vi "LogScales.vi"() -> ()   [LabVIEW 2013]
uses:
  <vilib>/Heliosphere Research LLC/Advanced Plotting Toolkit/api_core/NewPlotScales.ctl
  <vilib>/Heliosphere Research LLC/Advanced Plotting Toolkit/api_plotting/LineProperties.ctl
  <vilib>/Heliosphere Research LLC/Advanced Plotting Toolkit/properties/Line.ctl
  <vilib>/Heliosphere Research LLC/Advanced Plotting Toolkit/properties/Line_Style.ctl
  <vilib>/Heliosphere Research LLC/Advanced Plotting Toolkit/typedefs/PlotColor.ctl
  <vilib>/Heliosphere Research LLC/Advanced Plotting Toolkit/properties/Marker.ctl
  <vilib>/Heliosphere Research LLC/Advanced Plotting Toolkit/properties/Marker_Style.ctl
  <vilib>/Heliosphere Research LLC/Advanced Plotting Toolkit/properties/Display.ctl
  <vilib>/Heliosphere Research LLC/Advanced Plotting Toolkit/Advanced Plotting Toolkit.lvlib
panel:
  in  "Y Axis Scale":T1
  in  "X Axis Scale":T1
  in  "Show Grid Lines":bool=TRUE
  out "Log Plot":picture
  # "Log Scales"
  # "When plotting data that spans several orders of magnitude, it's\noften useful to display the X or Y axes using a log scale.\n\nThe Toolkit provides two mechanisms for this.  Scales of type\n\"Log\" are displayed in the traditional fashion, using base 10.\nTry changing the Y scale, below.\n\nThe second mechanism is \"Symlog\" or symmetric log.  This\nscale type displays both positive and negative values; since\nzero cannot be displayed on a log scale, a small region around\nthe origin will use a linear scale.\n\nTry changing the X scale, below.  In Log mode, only positive\nvalues are displayed.  In Symlog mode, both positive and\nnegative values are displayed."
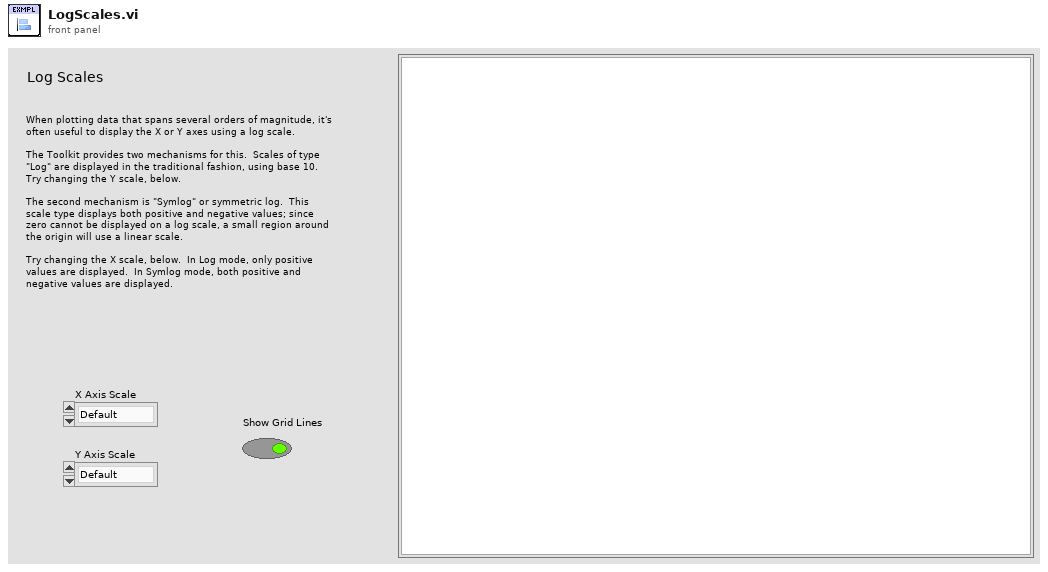
[diagram p1: front panel]
types:
  T1 = typedef "Advanced Plotting Toolkit.lvlib/NewPlotScales.ctl" = enum16{"Default", "Linear", "Log", "Symlog"}
  T2 = typedef "Advanced Plotting Toolkit.lvlib/Marker_Style.ctl" = enum16{"Automatic", "Circle", "Square", "Triangle", "Diamond", "Star", "Invisible"}
  T3 = typedef "Advanced Plotting Toolkit.lvlib/LineProperties.ctl" = cluster{"Line":T4, "Marker":T7, "Display":T8}
  T4 = typedef "Advanced Plotting Toolkit.lvlib/Line.ctl" = cluster{"Style":T5, "Color":T6, "Width":sgl}
  T5 = typedef "Advanced Plotting Toolkit.lvlib/Line_Style.ctl" = enum16{"Automatic", "Solid", "Dashed", "Dotted", "Dash-dot", "Invisible"}
  T6 = typedef "Advanced Plotting Toolkit.lvlib/PlotColor.ctl" = u32
  T7 = typedef "Advanced Plotting Toolkit.lvlib/Marker.ctl" = cluster{"Style":T2, "Color":T6, "Size":dbl}
  T8 = typedef "Advanced Plotting Toolkit.lvlib/Display.ctl" = cluster{"Alpha":dbl, "Z Order":dbl}
  T9 = typedef "Advanced Plotting Toolkit.lvlib/PlotID.ctl" = i32
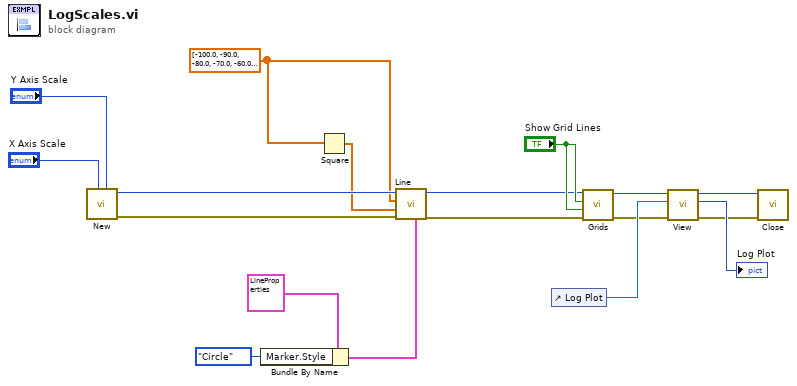
[diagram p0: block diagram]
diagram:
  w9 = dbl[] [-100.0, -90.0, -80.0, -70.0, -60.0, -50.0, -40.0, -30.0, -20.0, -10.0, 0.0, 10.0, 20.0, 30.0, 40.0, 50.0, 60.0, 70.0, 80.0, 90.0, 100.0] ("x+y")
  n1 = call <vilib>:"New.vi"("Y Axis Scale"="Y Axis Scale", "X Axis Scale"="X Axis Scale") -> ("error out"=w14:errorcluster, "Plot ID"=w15:T9)  [unwired: 8 in]
  n2 = Bundle By Name(cluster=T3 {"Line"={"Style"=enum."Automatic", "Color"=2147483647, "Width"=nan}, "Marker"={"Style"=enum."Automatic", "Color"=2147483647, "Size"=nan}, "Display"={"Alpha"=nan, "Z Order"=nan}} ("Line Plot Properties"), "Marker.Style"=Marker_Style."Circle") -> (w12:T3)
  n3 = Square(x=w9) -> (x^2=w10:dbl[])
  n4 = call <vilib>:"Line.vi"("Properties"=w12, "error in (no error)"=w14, "Y Data"=w10, "X Data"=w9, "Plot ID"=w15) -> ("error out"=w4:errorcluster, "Plot ID out"=w5:T9)  [unwired: 5 in]
  n5 = control-ref of="Log Plot"() -> (w18:refnum<vi>)
  n6 = call <vilib>:"Grids.vi"("error in (no error)"=w4, "Y Grid Lines (T)"="Show Grid Lines", "X Grid Lines (T)"="Show Grid Lines", "Plot ID"=w5) -> ("error out"=w7:errorcluster, "Plot ID Out"=w8:T9)  [unwired: 6 in]
  n7 = call <vilib>:"View.vi"("error in (no error)"=w7, "Ref for Sizing"=w18, "Plot ID"=w8) -> ("error out"=w1:errorcluster, "Picture"=→"Log Plot":picture, "Plot ID Out"=w16:T9)  [unwired: 6 in]
  n8 = call <vilib>:"Close.vi"("error in (no error)"=w1, "Plot ID"=w16) -> ()  [unwired: 9 in, 1 out]
